vi "Compute Double Buffer Length.vi"(2 "Duration (ms)":dbl, 3 "Sampling rate (Hz)":dbl) -> (0 "Double buffer length":i32, 1 "Sampling rate (out)":dbl)   [LabVIEW 2015]
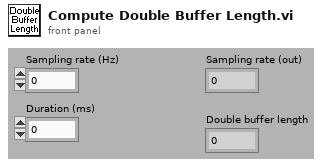
[diagram p1: front panel]
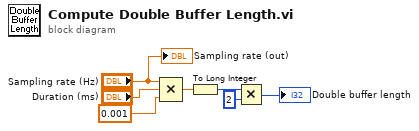
[diagram p0: block diagram]
diagram:
  n1 = Compound Arithmetic op=MULTIPLY("Sampling rate (Hz)", "Duration (ms)", 0.001) -> (w7:dbl)
  n2 = To Long Integer(number=w7) -> (32bit integer=w5:i32)
  n3 = Multiply(x=w5, y=2) -> (x*y=→"Double buffer length":i32)
  "Sampling rate (out)" <- "Sampling rate (Hz)"
